vi "DAQ_CollectDataQueueCreat.vi"(0 "reference in":refnum<class "DAQ_Base.lvclass">, 5 "error in (no error)":errorcluster) -> (14 "reference out":refnum<class "DAQ_Base.lvclass">, 19 "error out":errorcluster)   [LabVIEW 2020, in "DAQ.lvlib" / "DAQ_Base.lvclass"]
uses:
  DAQ_Base.lvclass
panel:
  out "CollectDataQueue":refnum<queue>
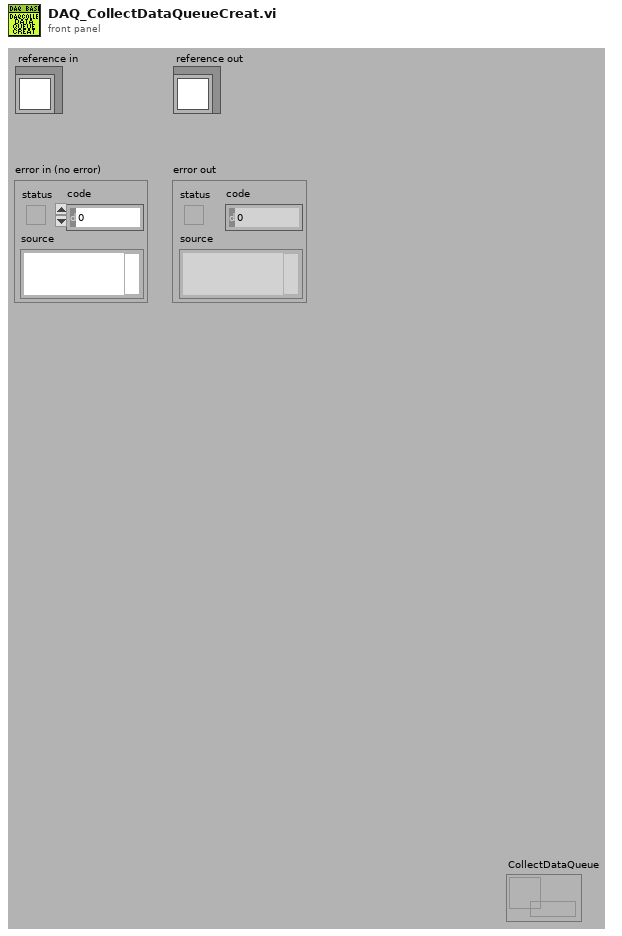
[diagram p1: front panel]
types:
  T1 = typedef "DAQ.lvlib/DAQ_Base.lvclass/ObjectAttributesRef.ctl" = refnum<data-value>
  T2 = typedef "DAQ.lvlib/DAQ_Base.lvclass/ObjectAttributes.ctl" = cluster{"MyAttribute":dbl, "RootPath":path, "DAQSettings":T3, "DaqCollector":cluster{"CollectDataQueue":refnum<queue>, "ArryDataCollectorChannel":T9[], "RealTimeValues":dbl[]}, "CollectorChannelEnable":bool[]}
  T3 = typedef "DAQ.lvlib/DAQ_Base.lvclass/DAQSettings.ctl" = cluster{"SampleSettings":T4, "AI_ChannelSettings":T5, "AO_ChannelSettings":T7, "Cnt_ChannelSettings":T8}
  T4 = typedef "DAQ.lvlib/DAQ_Base.lvclass/SampleSettings.ctl" = cluster{"samples per channel":i32, "SampleRate":dbl, "TansMaxLength":dbl, "ReadTimeOut":dbl, "时钟源":tag}
  T5 = typedef "DAQ.lvlib/DAQ_Base.lvclass/AI_ChannelSettings.ctl" = cluster{"AI_SettingsArry":cluster{"DeviceName":tag, "physical channels":tag, "AssignName":string, "输入信号类型":T6, "Max_value":dbl, "Min_value":dbl, "单位":i32, "shunt resistor location":i32, "external shunt resistor value":dbl, "标定系数":cluster{"Scale":dbl, "Offset":dbl}}[]}
  T6 = typedef "AI信号类型.ctl" = i32
  T7 = typedef "DAQ.lvlib/DAQ_Base.lvclass/AO_ChannelSettings.ctl" = cluster{"布尔":bool}
  T8 = typedef "DAQ.lvlib/DAQ_Base.lvclass/Cnt_ChannelSettings.ctl" = cluster{"Cnt_ChannelSettings":cluster{"类型":enum16{"Linear", "Rotate"}, "CounterNbr":tag, "AssignName":string, "单位":u16, "decoding type":u16, "PPR_DistancePerPulse":dbl, "Initial Position ":dbl, "z index enable":bool, "z index phase":i32, "source":tag}[]}
  T9 = typedef "DAQ.lvlib/DAQ_Base.lvclass/DataCollector.ctl" = cluster{"DataCollectArry":dbl[][], "Update":bool}
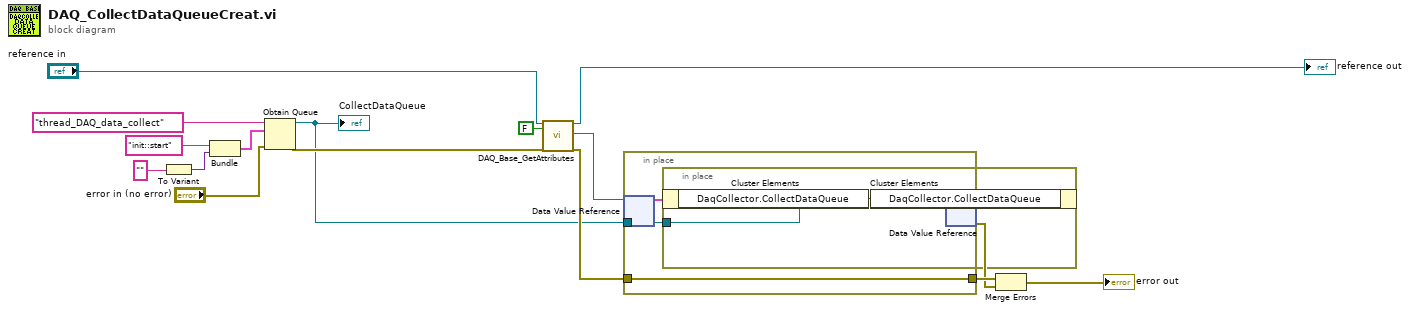
[diagram p0: block diagram]
diagram:
  n1 = To Variant(anything="") -> (Variant=w15:variant)
  n2 = Bundle("init::start", "Variant"=w15) -> (w13:cluster{string, "Variant":variant})  [unwired: 1 in]
  n3 = Obtain Queue(name (unnamed)="thread_DAQ_data_collect" ("名称（未命名）"), element data type=w13, error in (no error)="error in (no error)") -> (queue out=w2:refnum<queue>, error out=w3:errorcluster)  [unwired: 2 in, 1 out]
  "CollectDataQueue" <- w2
  n4 = call "DAQ_Base_GetAttributes.vi"("reference in"="reference in", "return data? (T)"=FALSE, "error in (no error)"=w3) -> ("reference out"=→"reference out":refnum<class "DAQ_Base.lvclass">, "attributes ref"=w7:T1, "error out"=w9:errorcluster)  [unwired: 13 in, 1 out]
  n5 = in-place {
    in-place-border: w9 -> [w18]
    in-place-border: [w18] -> w10
    in-place-border: w2 -> [w17]
    n6 = in-place-dvr #1(w7) -> (w19:T2)  [unwired: 1 out]
    n7 = in-place {
      in-place-border: w17 -> [w21]
      n8 = in-place-cluster #2(w19) -> ()  [unwired: 1 out]
      n9 = in-place-cluster #2("DaqCollector.CollectDataQueue"=w21) -> (w20:T2)
    }
    n10 = in-place-dvr #1(w20) -> (w8:errorcluster)  [unwired: 1 out]
  }
  n11 = Merge Errors(w10, w8) -> (→"error out":errorcluster)
